vi "Extend.vi"(0 "Ball":T1, 3 "ignoreBall?":bool, 4 "our_robots":T2[](array[typedef]), 5 "Goal":dbl[](array[numeric]), 6 "Step":dbl, 7 "Initial State":dbl[](array[numeric]), 8 "enemy_robots":T2[](array[typedef]), 9 "Robot in":T2={"id"=0, "function"=enum."Attacker", "x"=0.0, "y"=0.0, "orientation"=0.0, "v_tangent"=0.0, "v_normal"=0.0, "v_ang"=0.0, "kick_x"=0.0, "kick_z"=0.0, "dribble"=FALSE, "Timestamp"=timestamp(0 s since 1904-01-01), "estimatives"={"est_v_tangent"=0.0, "est_v_normal"=0.0, "est_vx"=0.0, "est_vy"=0.0, "Pos Robot Est"=[]}, "dest_x_kick"=0.0, "dest_y_kick"=0.0, "Gap Coord"=[], "States"=enum."GoToTangent", "Path "=[], "Path  Smooth"=[], "Dest"=[], "vx_desired"=0.0, "vy_desired"=0.0}, 10 "Target":dbl[](array[numeric]), 11 "Nearest":dbl[](array[numeric])) -> (2 "New State":dbl[](array[numeric]))   [LabVIEW 2018]
uses:
  Vision_class/Old vision/Controls/AI Robot.ctl
  Vision_class/Old vision/Controls/Functions Enum.ctl
  Vision_class/Old vision/Controls/AttackerStates.ctl
  Vision_class/Old vision/Controls/PathDests.ctl
  Vision_class/Old vision/Controls/PathDest.ctl
  Vision_class/Old vision/SSL Detection Frame Simple Estimator Cameras VelCmd Folder/Core/AI Ball.ctl
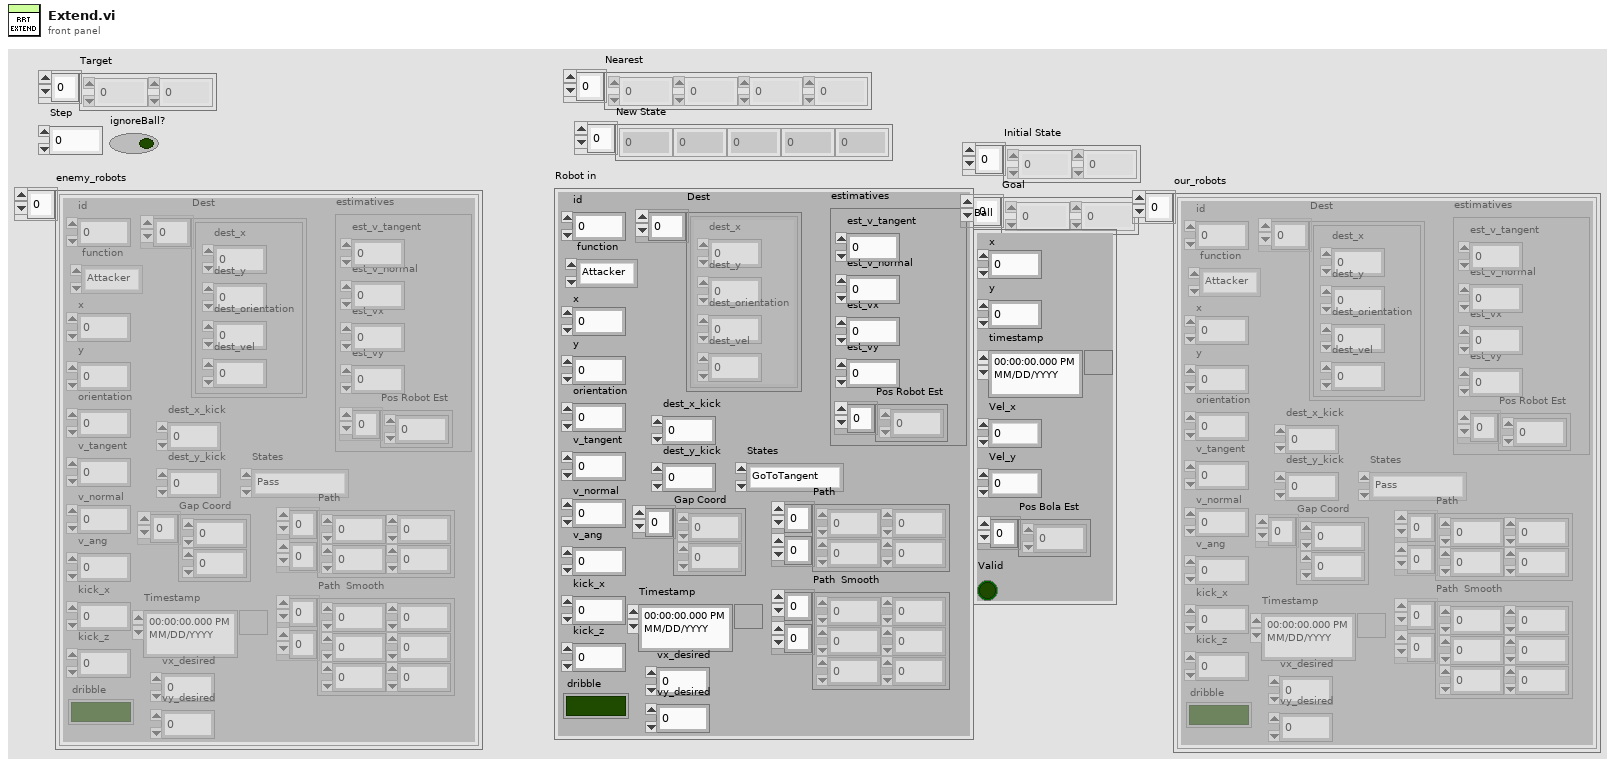
[diagram p1: front panel]
types:
  T1 = typedef "AI Ball.ctl" = cluster{"x":dbl, "y":dbl, "timestamp":timestamp, "Vel_x":dbl, "Vel_y":dbl, "Pos Bola Est":dbl[], "Valid":bool}
  T2 = typedef "AI Robot.ctl" = cluster{"id":u32, "function":T3, "x":dbl, "y":dbl, "orientation":dbl, "v_tangent":dbl, "v_normal":dbl, "v_ang":dbl, "kick_x":dbl, "kick_z":dbl, "dribble":bool, "Timestamp":timestamp, "estimatives":cluster{"est_v_tangent":dbl, "est_v_normal":dbl, "est_vx":dbl, "est_vy":dbl, "Pos Robot Est":dbl[]}, "dest_x_kick":dbl, "dest_y_kick":dbl, "Gap Coord":dbl[], "States":T4, "Path ":dbl[][], "Path  Smooth":dbl[][], "Dest":T5, "vx_desired":dbl, "vy_desired":dbl}
  T3 = typedef "Functions Enum.ctl" = enum16{"2nd Striker", "Attacker", "Goalie", "Defender", "Striker", "Goto 0", "Dummy", "Kicker", "ZigZag 0", "ZigZag 1", "ZigZag 2", "ZigZag 3", "ZigZag 4", "ZigZag 5", "ZigZag 6", "ZigZag 7", "ZigZag 8", ""}
  T4 = typedef "AttackerStates.ctl" = enum16{"Pass", "GoToTangent", "BallGetting", "GoToKick", ""}
  T5 = typedef "PathDests.ctl" = T6[]
  T6 = typedef "PathDest.ctl" = cluster{"dest_x":dbl, "dest_y":dbl, "dest_orientation":dbl, "dest_vel":dbl}
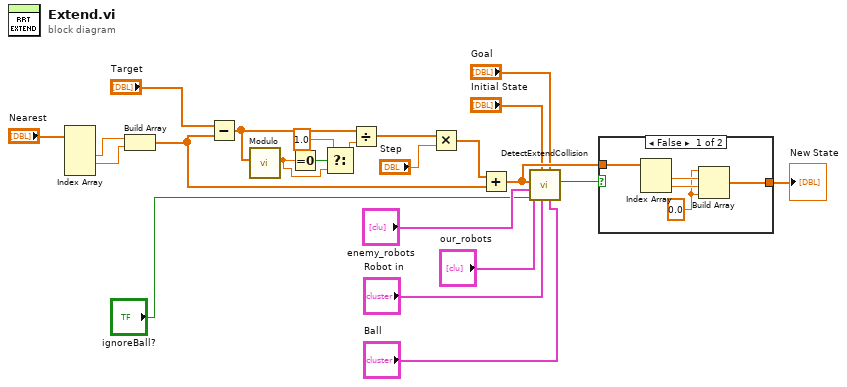
[diagram p0: block diagram]
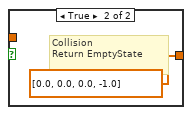
[diagram p2: hidden frame]
diagram:
  n1 = Index Array(array="Nearest") -> (element #2=w13:dbl, element #3=w12:dbl)  [unwired: 4 in, 2 out]
  n2 = Build Array(w13, w12) -> (w11:dbl[])
  n3 = Subtract(x="Target", y=w11) -> (x-y=w22:dbl[])
  n4 = call "Modulo.vi"("2D vector"=w22) -> ("Modulo"=w7:dbl)  [unwired: 10 in]
  n5 = Equal To 0?(x=w7) -> (x = 0?=w9:bool)
  n6 = Select(t=1.0, s=w9, f=w7) -> (s? t:f=w10:dbl)
  n7 = Divide(x=w22, y=w10) -> (x/y=w21:dbl[])
  n8 = Multiply(x=w21, y="Step") -> (x*y=w19:dbl[])
  n9 = Add(x=w19, y=w11) -> (x+y=w16:dbl[])
  n10 = call "DetectExtendCollision.vi"("Ball"="Ball", "Goal"="Goal", "Robot in"="Robot in", "Initial State"="Initial State", "ignoreBall?"="ignoreBall?", "enemy_robots"="enemy_robots", "Point"=w16, "our_robots"="our_robots") -> ("Collision"=w17:bool)  [unwired: 3 in]
  n11 = case shown="False" w17 {
    tunnel: [w24 dbl[] [0.0, 0.0, 0.0, -1.0] ("Nearest")] -> w15
    tunnel: w16 -> [w28 _]
    frame False {
      w25 = 0.0 ("element")
      n12 = Index Array(array=w28) -> (element #1=w27:dbl, element #2=w26:dbl)  [unwired: 2 in]
      n13 = Build Array(w25, w27, w26, w25) -> (w24:dbl[])
    }
    frame True {
      # "Collision\nReturn EmptyState"
    }
  }
  "New State" <- w15
